vi "partsTracking.vi"(8 "error in (no error)":errorcluster, 11 "reference in":refnum<class "Project Panels.lvclass">=refnum) -> (0 "error out":errorcluster, 2 "saved?":bool, 3 "reference out":refnum<class "Project Panels.lvclass">)   [LabVIEW 2015, in "Project Panels.lvclass"]
uses:
  Project Panels.lvclass
  <vilib>/Utility/miscctls.llb/LVRowAndColumnTypeDef.ctl
  stateItem.ctl
  SYS/PartsTracking Controller_class/PartsTracking Controller.lvclass
  SYS/Notification Controller_class/Notification Controller.lvclass
panel:
  out "Cell Position":T1={"Row"=0, "Column"=4}
  out "title":string="Cosmed Asia Pacific - Parts Tracking"
  in  "partsTracking":string[][](table)
  out "statuBar":string="Stoped from User"
  in  "Save":bool
  in  "Stop Button":bool
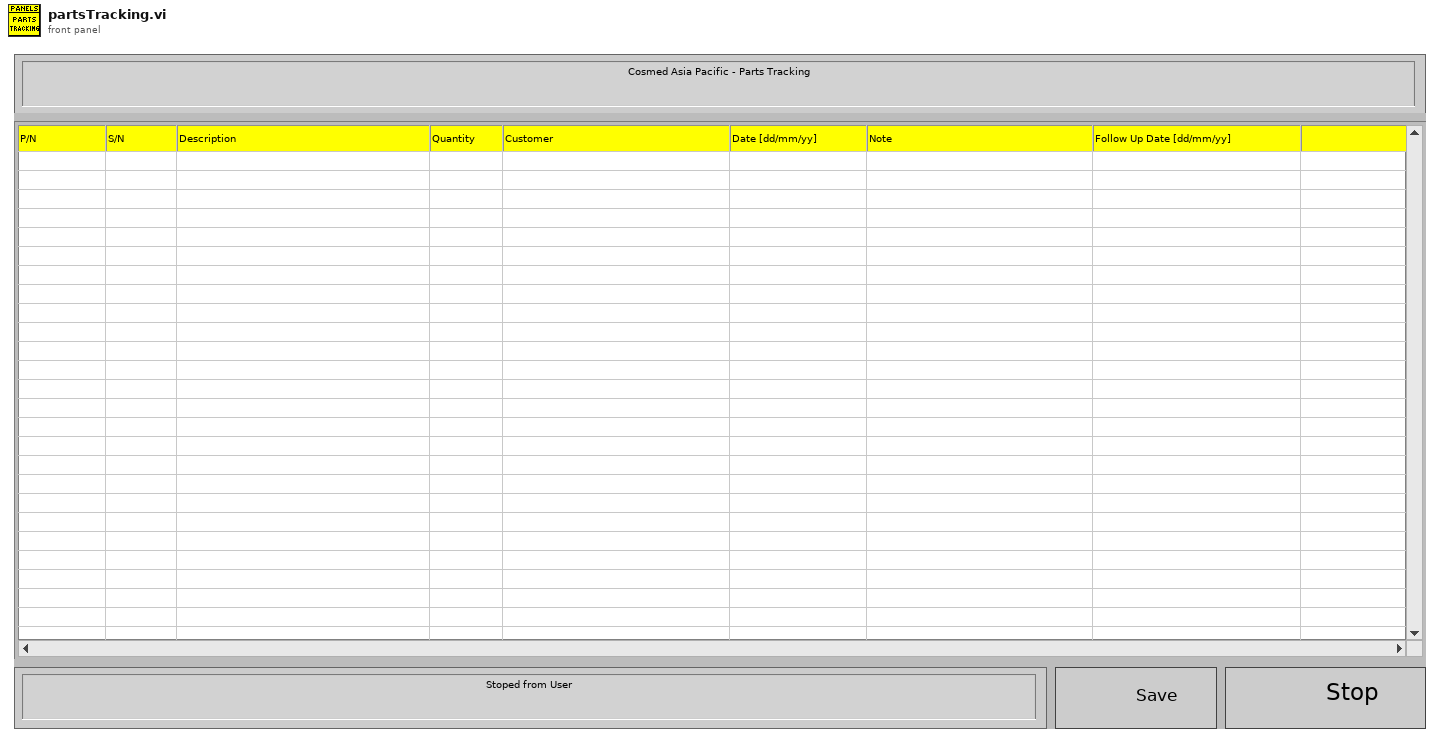
[diagram p1: front panel]
types:
  T1 = typedef "LVRowAndColumnTypeDef.ctl" = cluster{"Row":i32, "Column":i32}
  T2 = typedef "Project Panels.lvclass/stateItem.ctl" = enum16{"initiate", "waitEvent", "save", "search", "UploadFile", "nextItems", "stop"}
  T3 = typedef "Project Panels.lvclass/ObjectAttributesRef.ctl" = refnum<data-value>
  T4 = typedef "Project Panels.lvclass/ObjectAttributes.ctl" = cluster{"MyAttribute":dbl, "device_controller_ref":refnum<class "Devices Controller.lvclass">, "file_controller_ref":refnum<class "File Controller.lvclass">, "item_controller_ref":refnum<class "Items Controller.lvclass">, "item_tables":cluster{"checkIN":string[][], "checkOUT":string[][], "storage":string[][]}, "quickbook_table":cluster{"notes":string[][]}, "notification_controller_ref":refnum<class "Notification Controller.lvclass">, "partstracking_controller_ref":refnum<class "PartsTracking Controller.lvclass">, "product_tables":cluster{"k4b2":string[][], "fitmate":string[][], "RMR":string[][], "CPET":string[][], "BP":string[][], "PP":string[][], "k5":string[][], "bb-pft":string[][]}, "rowsColour":u32[]}
  T5 = typedef "LVPoint32TypeDef.ctl" = cluster{"Horizontal":i32, "Vertical":i32}
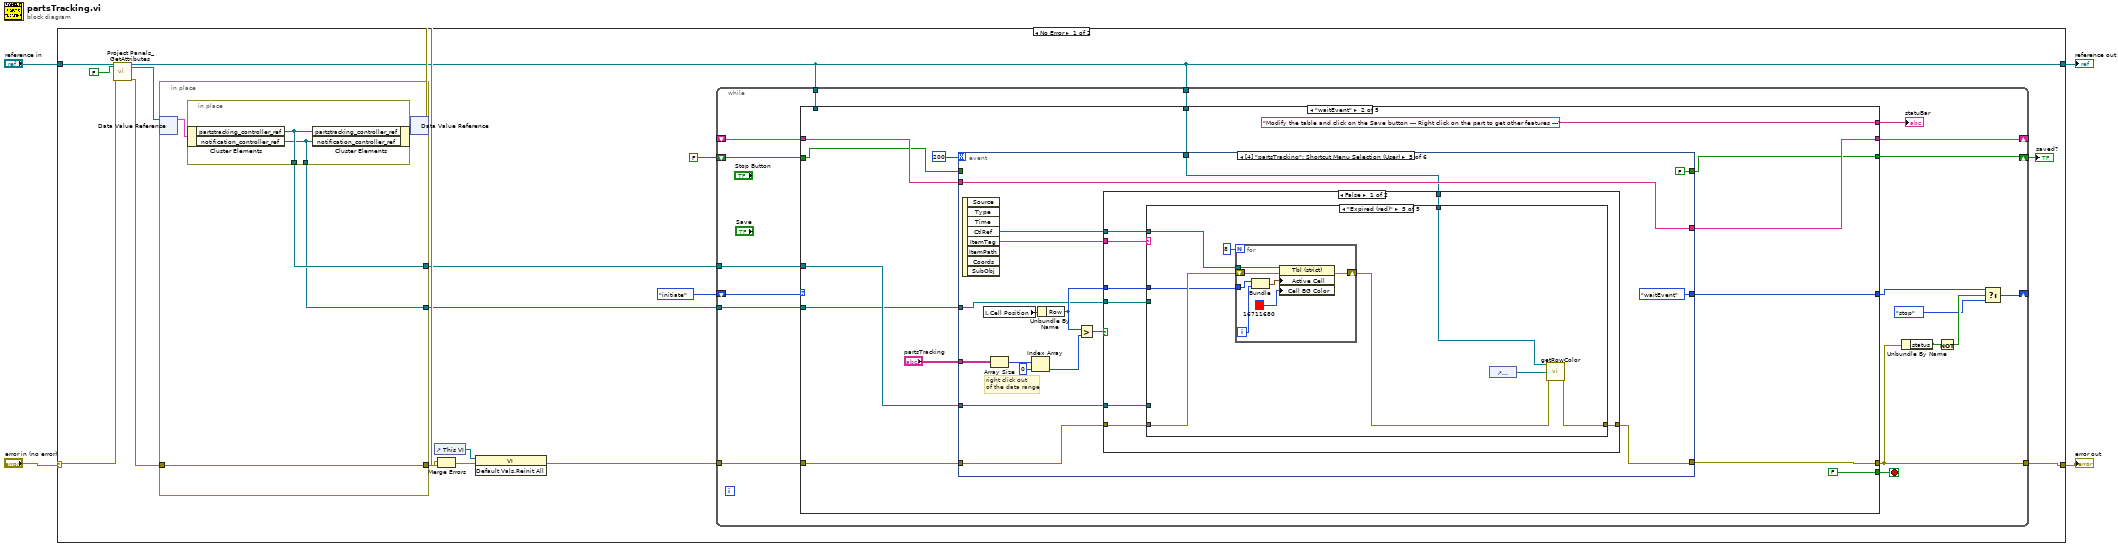
[diagram p0: block diagram]
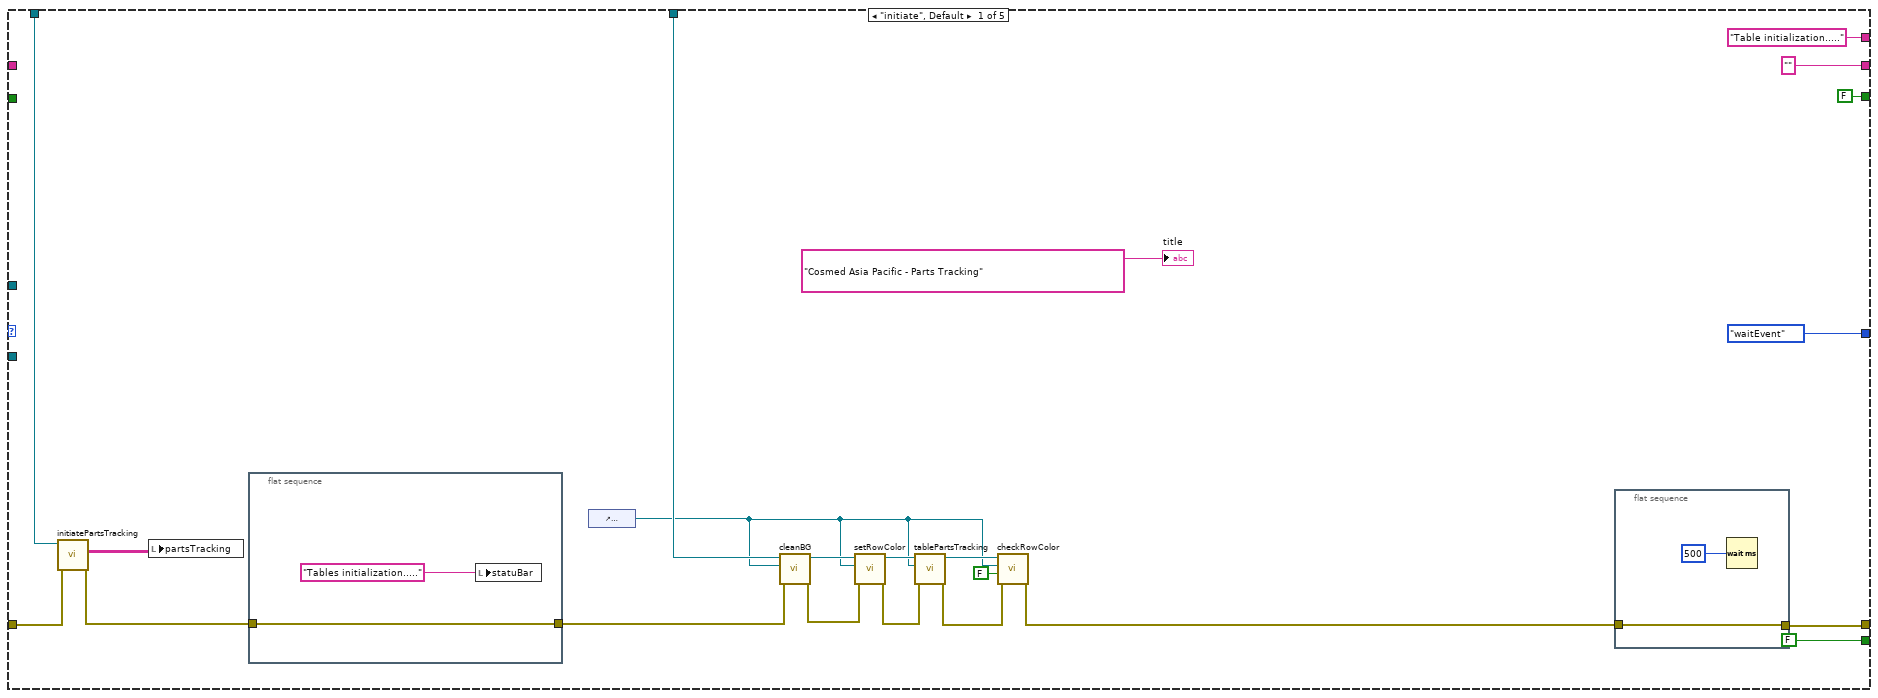
[diagram p2: hidden frame]
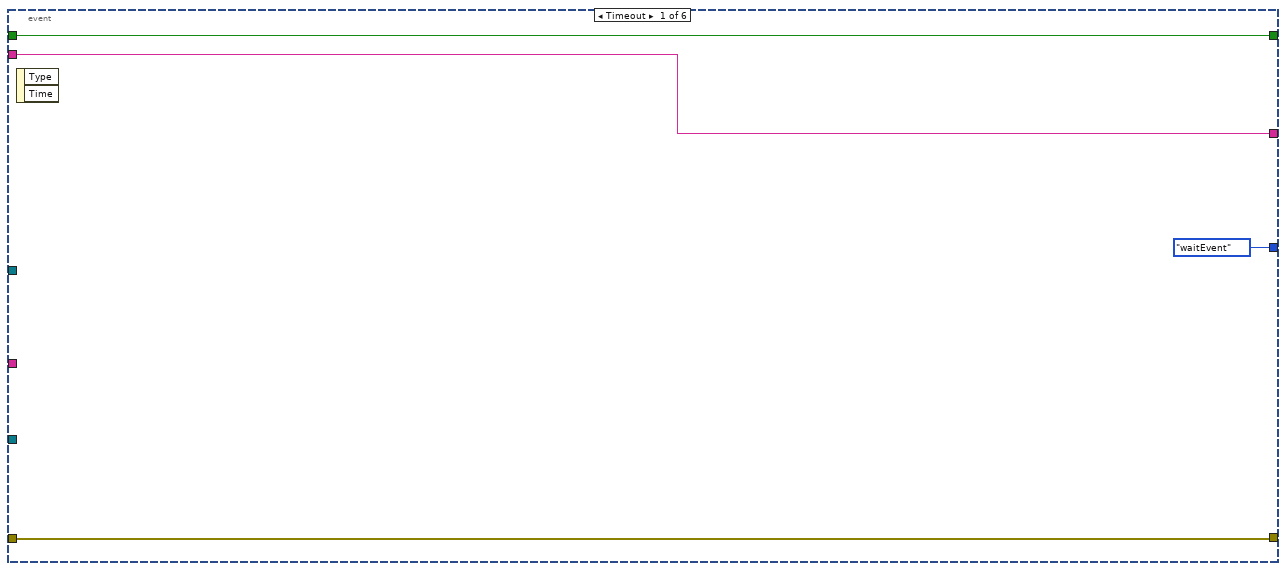
[diagram p3: hidden frame]
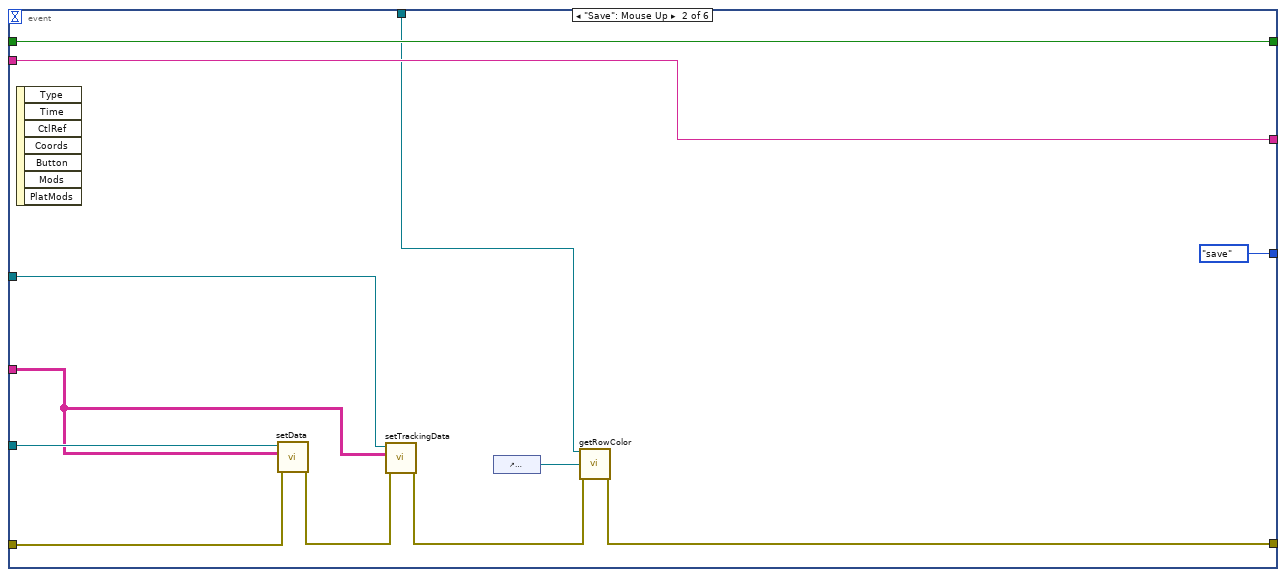
[diagram p4: hidden frame]
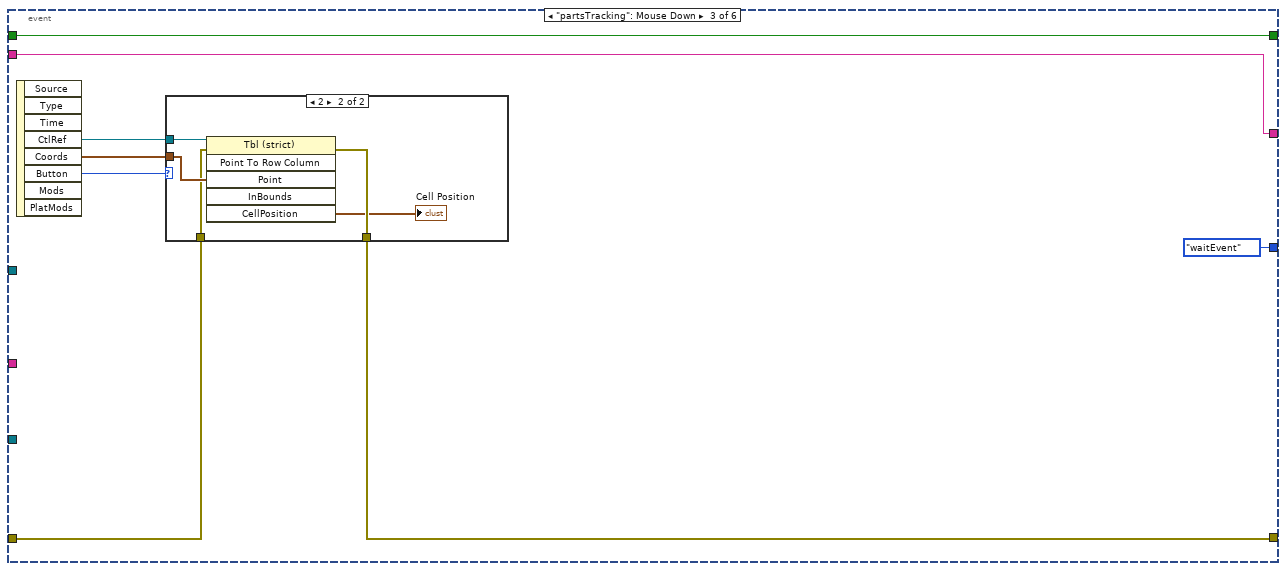
[diagram p5: hidden frame]
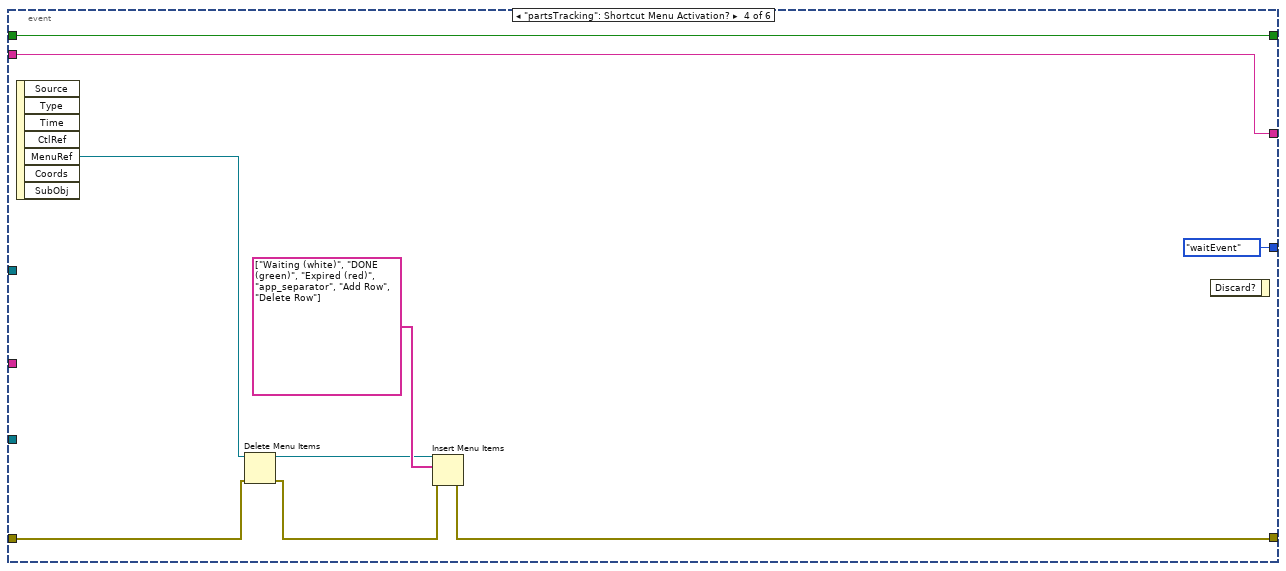
[diagram p7: hidden frame]
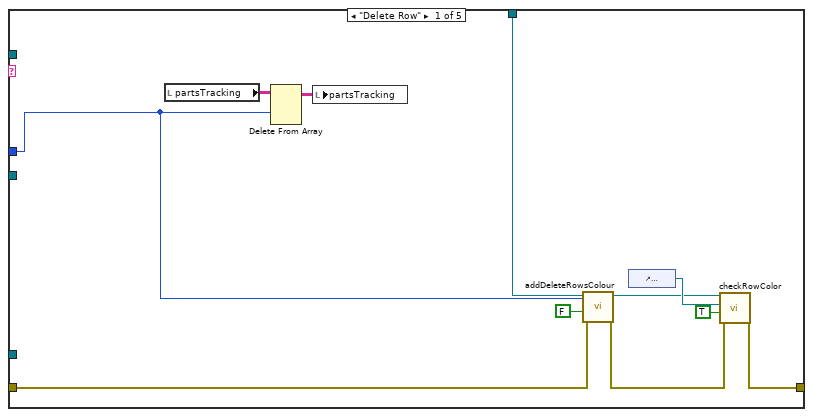
[diagram p8: hidden frame]
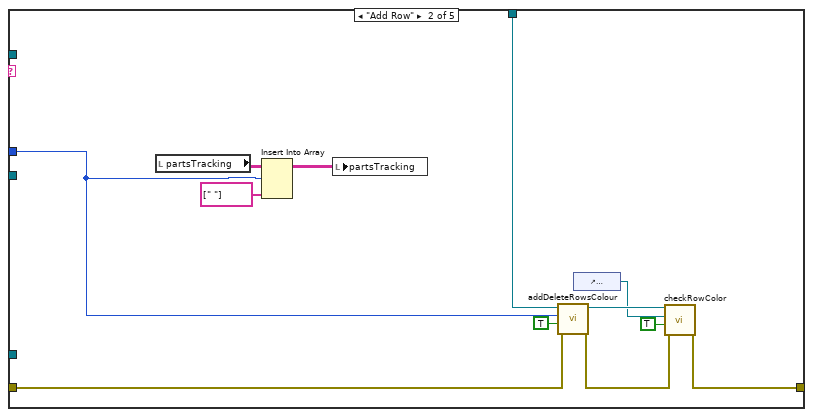
[diagram p9: hidden frame]
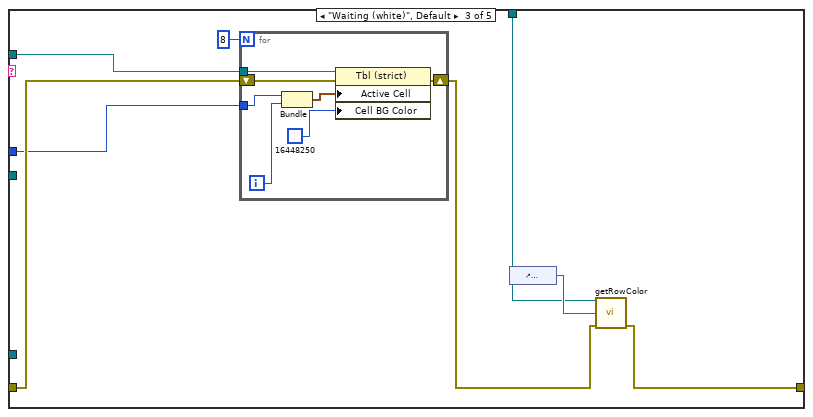
[diagram p10: hidden frame]
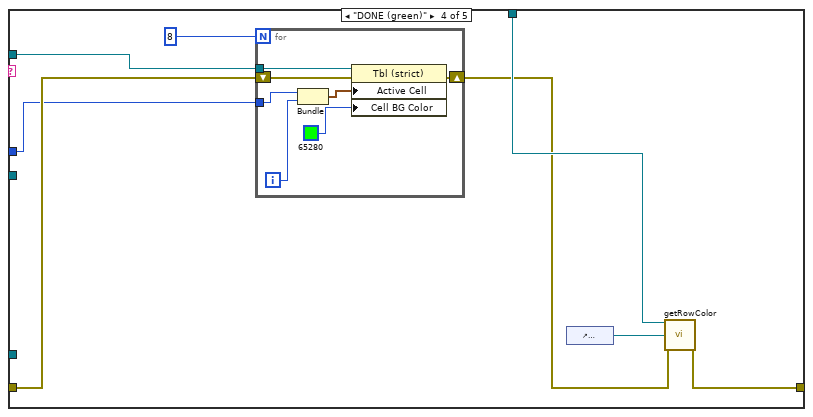
[diagram p11: hidden frame]
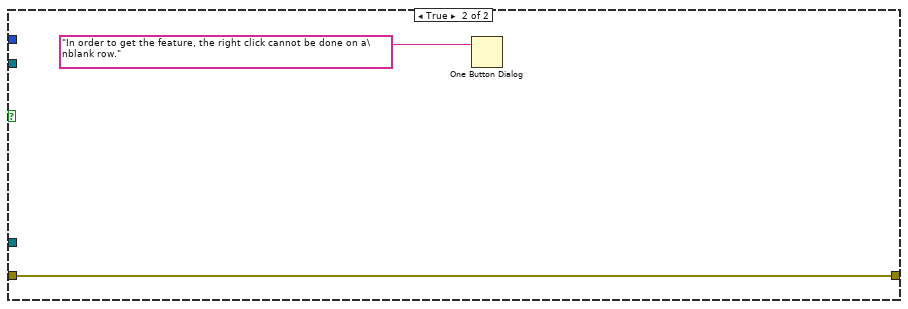
[diagram p12: hidden frame]
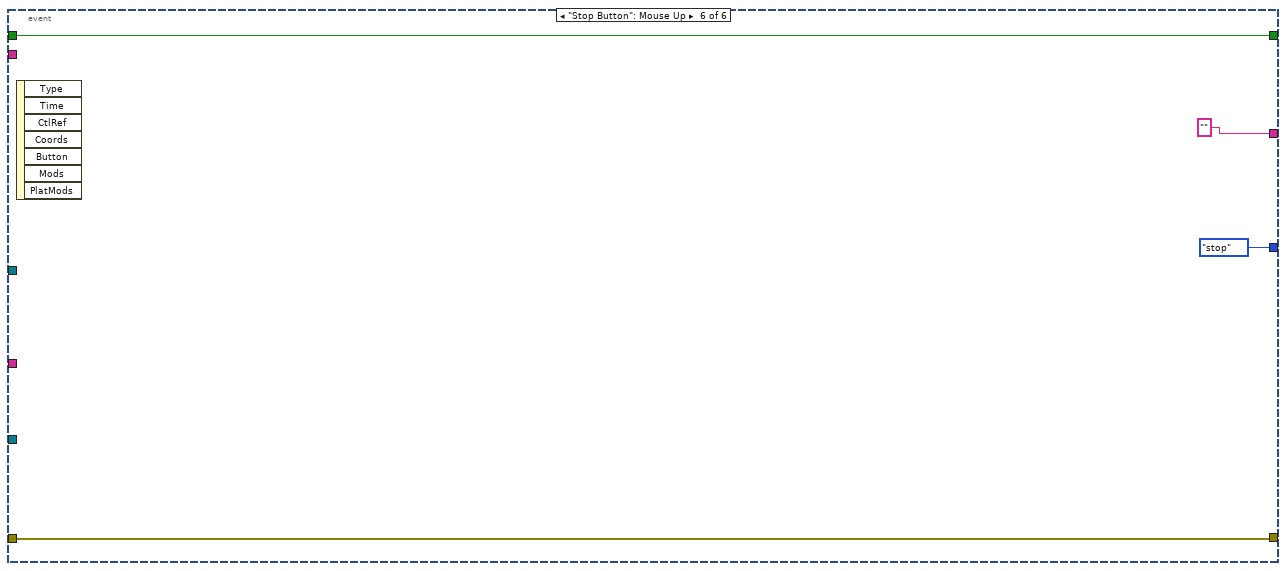
[diagram p13: hidden frame]
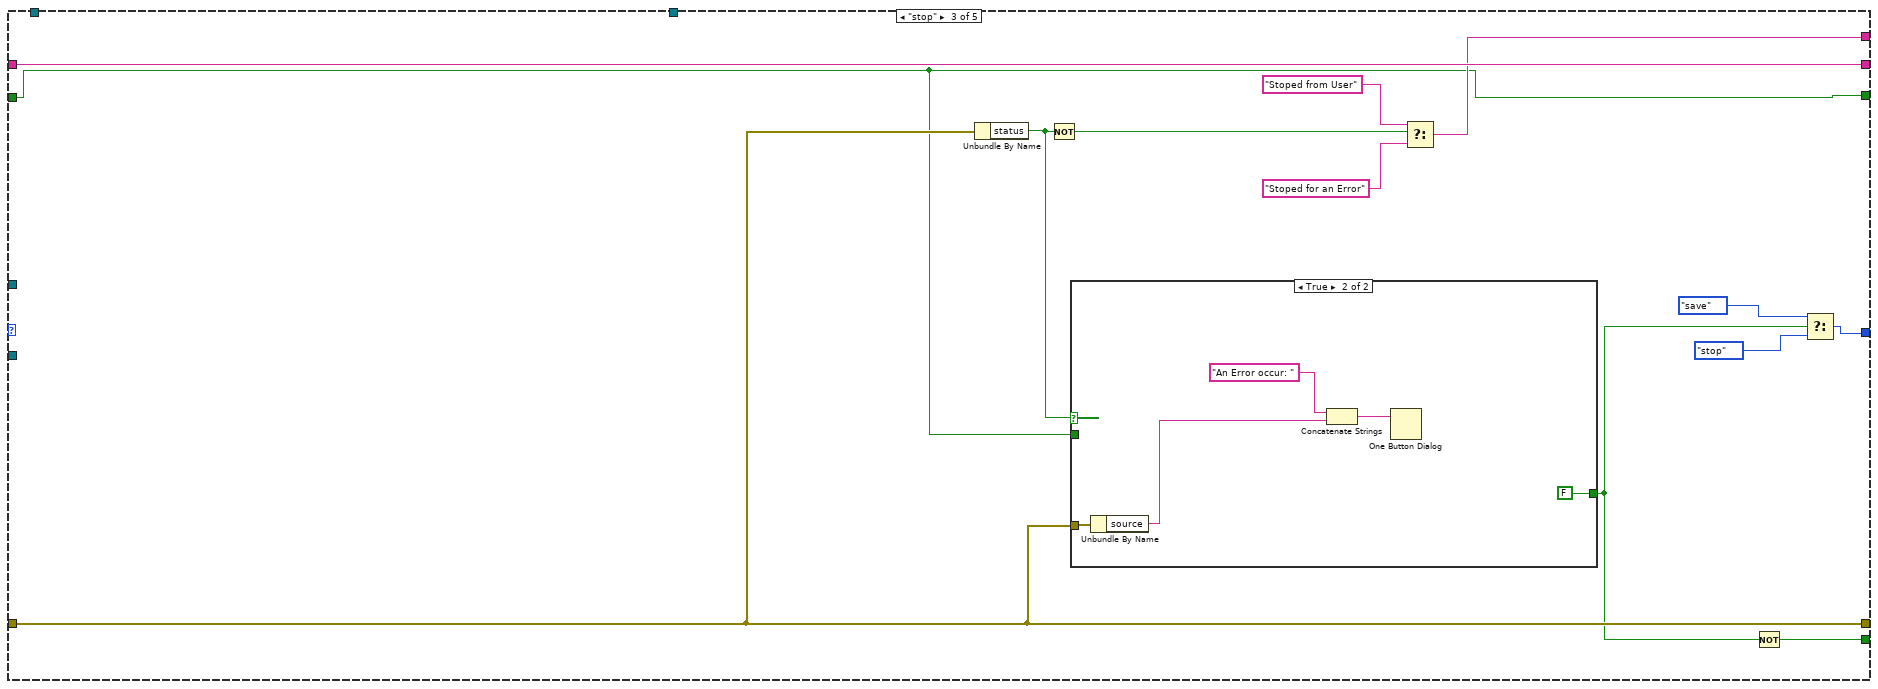
[diagram p14: hidden frame]
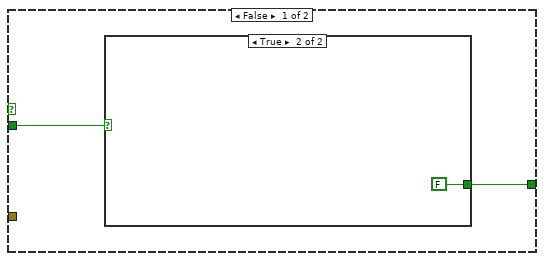
[diagram p15: hidden frame]
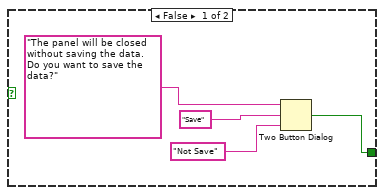
[diagram p16: hidden frame]
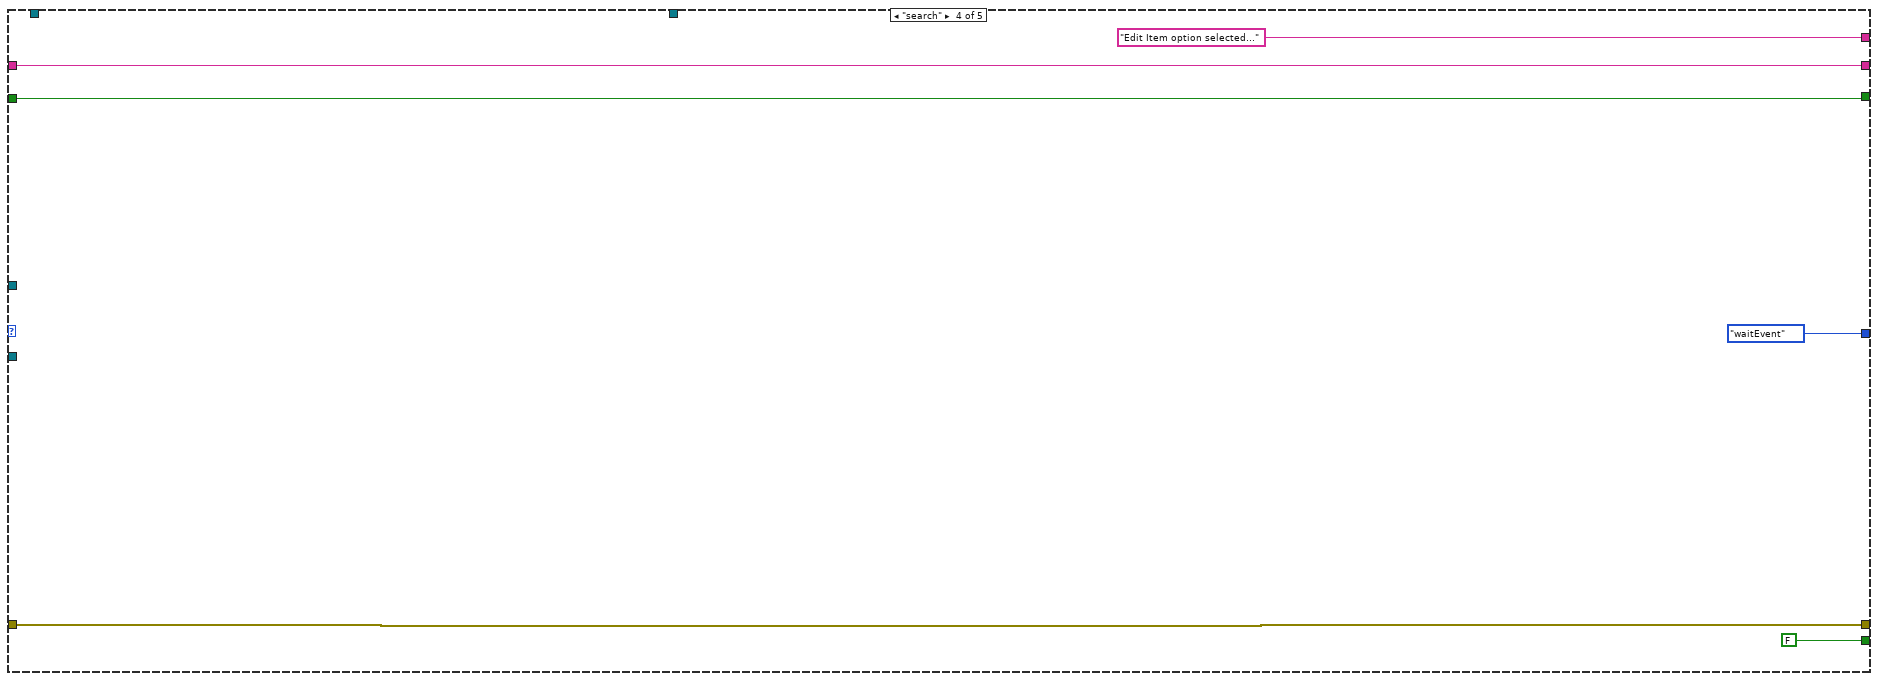
[diagram p17: hidden frame]
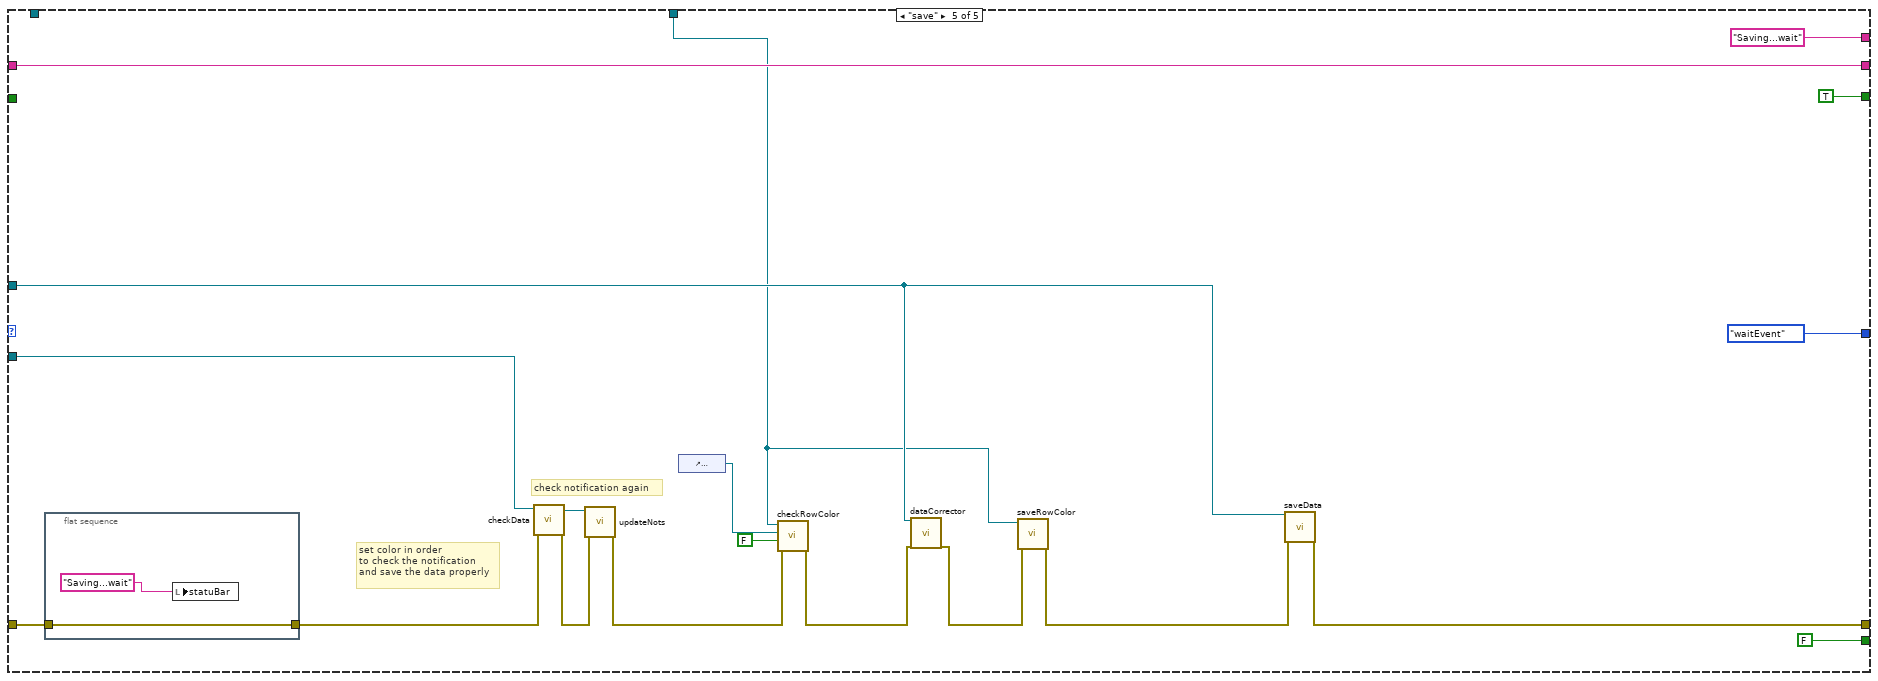
[diagram p18: hidden frame]
diagram:
  n1 = case shown="No Error" "error in (no error)" {
    selector: "error in (no error)" -> [w17 w278]
    tunnel: [w14 w278] -> w3
    tunnel: [w12 w277] -> w1
    tunnel: "reference in" -> [w19 w277]
    frame No Error {
      n2 = call "Project Panels_GetAttributes.vi"("reference in"=w19, "return data? (T)"=FALSE, "error in (no error)"=w17) -> ("reference out"=w12:refnum<class "Project Panels.lvclass">, "attributes ref"=w15:T3, "error out"=w16:errorcluster)  [unwired: 13 in, 1 out]
      n3 = in-place {
        in-place-border: w16 -> [w272]
        in-place-border: [w272] -> w20
        in-place-border: [w271] -> w10
        in-place-border: [w270] -> w6
        n4 = in-place-dvr #1(w15) -> (w273:T4)  [unwired: 1 out]
        n5 = in-place {
          in-place-border: [w276] -> w271
          in-place-border: [w275] -> w270
          n6 = in-place-cluster #2(w273) -> ("partstracking_controller_ref"=w276:refnum<class "PartsTracking Controller.lvclass">, "notification_controller_ref"=w275:refnum<class "Notification Controller.lvclass">)
          n7 = in-place-cluster #2("partstracking_controller_ref"=w276, "notification_controller_ref"=w275) -> (w274:T4)
        }
        n8 = in-place-dvr #1(w274) -> (w21:errorcluster)  [unwired: 1 out]
      }
      n9 = control-ref of="This VI"() -> (w11:refnum<vi>)
      n10 = Merge Errors(w20, w21) -> (w7:errorcluster)
      n11 = invoke class="VI" method="Default Vals.Reinit All"(reference=w11, error in=w7) -> (error out=w5:errorcluster)  [unwired: 1 in, 2 out]
      n12 = while {
        tunnel: w12 -> [w39]
        tunnel: w5 -> [w22]
        tunnel: [w37] -> w14
        shift-right: [w34] -> _
        shift-left: stateItem."initiate" ("state") -> [w38]
        shift-right: [w30] -> _
        shift-left: _ -> [w29]
        tunnel: w12 -> [w28]
        tunnel: w10 -> [w26]
        shift-right: [w24] -> w8
        shift-left: FALSE -> [w25]
        tunnel: w6 -> [w23]
        stop <- w32 stop-if-true
        n13 = case shown="\"waitEvent\"" w38 {
          tunnel: w39 -> [w45 w70 _ _ w251]
          tunnel: w22 -> [w54 w78 w221 w244 w263]
          tunnel: [w58 w73 w221 w244 w254] -> w37
          tunnel: [stateItem."waitEvent" ("state") w72 w223 stateItem."waitEvent" ("state") stateItem."waitEvent" ("state")] -> w35
          tunnel: [FALSE FALSE w218 FALSE FALSE] -> w32
          tunnel: ["Table initialization....." ("title") "Modify the table and click on the Save button --- Right click on the part to get other features ---" ("title") w227 "Edit Item option selected..." ("title") "Saving...wait" ("title")] -> w31
          tunnel: ["" w74 w230 w246 w265] -> w30
          tunnel: w29 -> [_ w75 w230 w246 w265]
          tunnel: w28 -> [w55 _ _ _ _]
          tunnel: w26 -> [_ w71 _ _ w257]
          tunnel: w25 -> [_ w68 w220 w243 _]
          tunnel: [FALSE w67 w220 w243 TRUE] -> w24
          tunnel: w23 -> [_ w69 _ _ w262]
          frame "initiate", Default {
            n14 = call "initiatePartsTracking.vi"("error in (no error)"=w54, "reference in"=w55) -> ("error out"=w53:errorcluster, "data"=w52:string[][])  [unwired: 7 in, 1 out]
            n15 = local write "partsTracking"(w52) -> ()
            n16 = flat-sequence {
              tunnel: w53 -> [w63]
              tunnel: [w63] -> w42
              frame #0 {
                n17 = local write "statuBar"("Tables initialization....." ("title")) -> ()
              }
            }
            n18 = control-ref of="partsTracking"() -> (w43:refnum<vi>)
            n19 = call "cleanBG.vi"("error in (no error)"=w42, "Table in"=w43, "reference in"=w45) -> ("error out"=w41:errorcluster, "reference out"=w44:refnum<class "Project Panels.lvclass">)  [unwired: 7 in]
            n20 = call "setRowColor.vi"("error in (no error)"=w41, "Table in"=w43, "reference in"=w44) -> ("error out"=w50:errorcluster, "reference out"=w51:refnum<class "Project Panels.lvclass">)  [unwired: 7 in]
            n21 = call "tablePartsTracking.vi"("error in (no error)"=w50, "Table in"=w43, "reference in"=w51) -> ("error out"=w48:errorcluster, "reference out"=w49:refnum<class "Project Panels.lvclass">)  [unwired: 7 in]
            n22 = call "checkRowColor.vi"("error in (no error)"=w48, "add/delete"=FALSE, "Table in"=w43, "reference in"=w49) -> ("error out"=w47:errorcluster)  [unwired: 6 in, 1 out]
            n23 = flat-sequence {
              tunnel: w47 -> [w65]
              tunnel: [w65] -> w58
              frame #0 {
                n24 = Wait (ms)(milliseconds to wait=u32 500) -> ()  [unwired: 1 out]
              }
            }
            "title" <- "Cosmed Asia Pacific - Parts Tracking" ("title")
          }
          frame "waitEvent" {
            n25 = event shown="[4] \"partsTracking\": Shortcut Menu Selection (User)" {
              selector: _ -> [_ _ _ _ _ _]
              dyn-events: _ -> [_ _ _ _ _ _]
              timeout: 200 -> [_ _ _ _ _ _]
              tunnel: w78 -> [w83 w93 w98 w116 w132 w217]
              tunnel: [w83 w85 w97 w113 w131 w217] -> w73
              tunnel: w75 -> [w82 w95 w101 w118 w135 _]
              tunnel: [w82 w95 w101 w118 w135 ""] -> w74
              tunnel: [stateItem."waitEvent" ("state") stateItem."save" ("state") stateItem."waitEvent" ("state") stateItem."waitEvent" ("state") stateItem."waitEvent" ("state") stateItem."stop" ("state")] -> w72
              tunnel: w71 -> [_ w92 _ _ w122 _]
              tunnel: w70 -> [_ w84 _ _ w119 _]
              tunnel: w69 -> [_ w90 _ _ w121 _]
              tunnel: w68 -> [w80 w89 w96 w110 _ w214]
              tunnel: [w80 w89 w96 w110 FALSE w214] -> w67
              tunnel: "partsTracking" -> [_ w88 _ _ w129 _]
              event Timeout {
                n26 = event-data() -> ()  [unwired: 1 in, 2 out]
              }
              event "Save": Mouse Up {
                n27 = event-data() -> ()  [unwired: 1 in, 7 out]
                n28 = call "setData.vi"("error in (no error)"=w93, "Data"=w88, "reference in"=w92) -> ("error out"=w91:errorcluster)  [unwired: 7 in, 1 out]
                n29 = call "setTrackingData.vi"("error in (no error)"=w91, "tracking_parts_data"=w88, "reference in"=w90) -> ("error out"=w86:errorcluster)  [unwired: 7 in, 1 out]
                n30 = control-ref of="partsTracking"() -> (w87:refnum<vi>)
                n31 = call "getRowColor.vi"("reference in"=w84, "Table in"=w87, "error in (no error)"=w86) -> ("error out"=w85:errorcluster)  [unwired: 11 in, 1 out]
              }
              event "partsTracking": Mouse Down {
                n32 = event-data() -> ("CtlRef"=w100:refnum<vi>, "Coords"=w99:T5, "Button"=w103:u16)  [unwired: 1 in, 5 out]
                n33 = case shown="2" w103 {
                  tunnel: w100 -> [_ w109]
                  tunnel: w99 -> [_ w108]
                  tunnel: w98 -> [w104 w107]
                  tunnel: [w104 w106] -> w97
                  frame 0, Default {
                  }
                  frame 2 {
                    n34 = invoke class="Tbl (strict)" method="Point To Row Column"(reference=w109, error in=w107, "Point"=w108) -> (error out=w106:errorcluster, "CellPosition"=→"Cell Position":T1)  [unwired: 3 in, 4 out]
                  }
                }
              }
              event "partsTracking": Shortcut Menu Activation? {
                n35 = event-data() -> ("MenuRef"=w115:refnum<k9>)  [unwired: 1 in, 6 out]
                n36 = Delete Menu Items(6:w116, 9:w115) -> (0:w114:errorcluster, 3:w111:refnum<k9>)  [unwired: 2 in]
                n37 = Insert Menu Items(6:w114, 8:string[] ["Waiting (white)", "DONE (green)", "Expired (red)", "app_separator", "Add Row", "Delete Row"] ("item names"), 9:w111) -> (0:w113:errorcluster)  [unwired: 3 in, 2 out]
                n38 = event-data() -> ()  [unwired: 2 in, 1 out]
              }
              event "partsTracking": Shortcut Menu Selection (User) {
                # "right click out\nof the data range"
                n39 = event-data() -> ("CtlRef"=w133:refnum<vi>, "ItemTag"=w134:string)  [unwired: 1 in, 6 out]
                n40 = local read "Cell Position"() -> (w126:T1)
                n41 = Array Size(array=w129) -> (size(s)=w128:i32[])
                n42 = Index Array(array=w128, index=0) -> (element=w125:i32)
                n43 = Unbundle By Name(w126) -> ("Row"=w123:i32)
                n44 = Greater?(x=w123, y=w125) -> (0:w124:bool)
                n45 = case shown="False" w124 {
                  tunnel: w134 -> [w143 _]
                  tunnel: w133 -> [w142 _]
                  tunnel: w132 -> [w141 w213]
                  tunnel: [w140 w213] -> w131
                  tunnel: w123 -> [w139 _]
                  tunnel: w122 -> [w138 _]
                  tunnel: w121 -> [w137 _]
                  tunnel: w119 -> [w136 _]
                  frame False {
                    n46 = case shown="\"Expired (red)\"" w143 {
                      tunnel: w142 -> [_ _ w174 w188 w203]
                      tunnel: w141 -> [w149 w161 w173 w187 w202]
                      tunnel: [w144 w157 w167 w182 w197] -> w140
                      tunnel: w139 -> [w150 w162 w171 w186 w201]
                      tunnel: w138 -> [_ _ _ _ _]
                      tunnel: w137 -> [_ _ _ _ _]
                      tunnel: w136 -> [w151 w163 w169 w184 w199]
                      frame "Delete Row" {
                        n47 = local read "partsTracking"() -> (w154:string[][])
                        n48 = Delete From Array(array=w154, index (row)=w150) -> (array with subset deleted=w153:string[][])  [unwired: 2 in, 1 out]
                        n49 = local write "partsTracking"(w153) -> ()
                        n50 = call "addDeleteRowsColour.vi"("error in (no error)"=w149, "Add?"=FALSE, "index"=w150, "reference in"=w151) -> ("error out"=w145:errorcluster, "reference out"=w146:refnum<class "Project Panels.lvclass">)  [unwired: 6 in]
                        n51 = control-ref of="partsTracking"() -> (w148:refnum<vi>)
                        n52 = call "checkRowColor.vi"("error in (no error)"=w145, "add/delete"=TRUE, "Table in"=w148, "reference in"=w146) -> ("error out"=w144:errorcluster)  [unwired: 6 in, 1 out]
                      }
                      frame "Add Row" {
                        n53 = local read "partsTracking"() -> (w166:string[][])
                        n54 = Insert Into Array(array=w166, index (row)=w162, new element=string[] [" "] ("new element/subarray")) -> (w164:string[][])  [unwired: 1 in]
                        n55 = local write "partsTracking"(w164) -> ()
                        n56 = call "addDeleteRowsColour.vi"("error in (no error)"=w161, "Add?"=TRUE, "index"=w162, "reference in"=w163) -> ("error out"=w158:errorcluster, "reference out"=w159:refnum<class "Project Panels.lvclass">)  [unwired: 6 in]
                        n57 = control-ref of="partsTracking"() -> (w156:refnum<vi>)
                        n58 = call "checkRowColor.vi"("error in (no error)"=w158, "add/delete"=TRUE, "Table in"=w156, "reference in"=w159) -> ("error out"=w157:errorcluster)  [unwired: 6 in, 1 out]
                      }
                      frame "Waiting (white)", Default {
                        n59 = for {
                          N: 8 -> [_]
                          tunnel: w174 -> [w181]
                          shift-right: [w179] -> w168
                          shift-left: w173 -> [w180]
                          tunnel: w171 -> [w177]
                          i -> [w176]
                          n60 = Bundle("Row"=w177, w176) -> (w175:cluster{"Row":i32, i32})  [unwired: 1 in]
                          n61 = property class="Tbl (strict)"(reference=w181, error in=w180, "Active Cell"=w175, "Cell BG Color"=u32 16448250) -> (error out=w179:errorcluster)  [unwired: 1 out]
                        }
                        n62 = control-ref of="partsTracking"() -> (w170:refnum<vi>)
                        n63 = call "getRowColor.vi"("reference in"=w169, "Table in"=w170, "error in (no error)"=w168) -> ("error out"=w167:errorcluster)  [unwired: 11 in, 1 out]
                      }
                      frame "DONE (green)" {
                        n64 = for {
                          N: 8 -> [_]
                          tunnel: w188 -> [w196]
                          shift-right: [w194] -> w183
                          shift-left: w187 -> [w195]
                          tunnel: w186 -> [w192]
                          i -> [w191]
                          n65 = Bundle("Row"=w192, w191) -> (w190:cluster{"Row":i32, i32})  [unwired: 1 in]
                          n66 = property class="Tbl (strict)"(reference=w196, error in=w195, "Active Cell"=w190, "Cell BG Color"=u32 65280) -> (error out=w194:errorcluster)  [unwired: 1 out]
                        }
                        n67 = control-ref of="partsTracking"() -> (w185:refnum<vi>)
                        n68 = call "getRowColor.vi"("reference in"=w184, "Table in"=w185, "error in (no error)"=w183) -> ("error out"=w182:errorcluster)  [unwired: 11 in, 1 out]
                      }
                      frame "Expired (red)" {
                        n69 = for {
                          N: 8 -> [_]
                          tunnel: w203 -> [w211]
                          shift-right: [w209] -> w198
                          shift-left: w202 -> [w210]
                          tunnel: w201 -> [w207]
                          i -> [w205]
                          n70 = Bundle("Row"=w207, w205) -> (w206:cluster{"Row":i32, i32})  [unwired: 1 in]
                          n71 = property class="Tbl (strict)"(reference=w211, error in=w210, "Active Cell"=w206, "Cell BG Color"=u32 16711680) -> (error out=w209:errorcluster)  [unwired: 1 out]
                        }
                        n72 = control-ref of="partsTracking"() -> (w200:refnum<vi>)
                        n73 = call "getRowColor.vi"("reference in"=w199, "Table in"=w200, "error in (no error)"=w198) -> ("error out"=w197:errorcluster)  [unwired: 11 in, 1 out]
                      }
                    }
                  }
                  frame True {
                    n74 = One Button Dialog(message="In order to get the feature, the right click cannot be done on a\nblank row.") -> ()  [unwired: 1 in, 1 out]
                  }
                }
              }
              event "Stop Button": Mouse Up {
                n75 = event-data() -> ()  [unwired: 1 in, 7 out]
              }
            }
          }
          frame "stop" {
            n76 = Unbundle By Name(w221) -> ("status"=w226:bool)
            n77 = Not(x=w226) -> (.not. x?=w225:bool)
            n78 = case shown="True" w226 {
              tunnel: w221 -> [_ w240]
              tunnel: [w232 FALSE ("Save")] -> w219
              tunnel: w220 -> [w231 _]
              frame False {
                n79 = case shown="True" w231 {
                  tunnel: [w235 FALSE ("Save")] -> w232
                  frame False {
                    n80 = Two Button Dialog(message="The panel will be closed without saving the data. Do you want to save the data?", 1:"Not Save" ("F button name (\"Cancel\")"), 2:"Save" ("T button name (\"OK\")")) -> (T button?=w235:bool)
                  }
                  frame True {
                  }
                }
              }
              frame True {
                n81 = Unbundle By Name(w240) -> ("source"=w239:string)
                n82 = Concatenate Strings("An Error occur: " ("message"), w239) -> (w242:string)
                n83 = One Button Dialog(message=w242) -> ()  [unwired: 1 in, 1 out]
              }
            }
            n84 = Select(t="Stoped from User" ("title"), s=w225, f="Stoped for an Error" ("title")) -> (s? t:f=w227:string)
            n85 = Not(x=w219) -> (.not. x?=w218:bool)
            n86 = Select(t=stateItem."save", s=w219, f=stateItem."stop" ("state")) -> (s? t:f=w223:T2)
          }
          frame "search" {
          }
          frame "save" {
            # "set color in order\nto check the notification\nand save the data properly"
            # "check notification again"
            n87 = flat-sequence {
              tunnel: w263 -> [w269]
              tunnel: [w269] -> w256
              frame #0 {
                n88 = local write "statuBar"("Saving...wait" ("title")) -> ()
              }
            }
            n89 = call "checkData.vi"("error in (no error)"=w256, "reference in"=w262) -> ("error out"=w260:errorcluster, "reference out"=w261:refnum<class "Notification Controller.lvclass">)  [unwired: 8 in]
            n90 = call "updateNots.vi"("error in (no error)"=w260, "reference in"=w261) -> ("error out"=w253:errorcluster)  [unwired: 8 in, 1 out]
            n91 = control-ref of="partsTracking"() -> (w258:refnum<vi>)
            n92 = call "checkRowColor.vi"("error in (no error)"=w253, "add/delete"=FALSE, "Table in"=w258, "reference in"=w251) -> ("error out"=w252:errorcluster)  [unwired: 6 in, 1 out]
            n93 = call "dataCorrector.vi"("reference in"=w257, "error in (no error)"=w252) -> ("error out"=w250:errorcluster)  [unwired: 16 in, 1 out]
            n94 = call "saveRowColor.vi"("error in (no error)"=w250, "reference in"=w251) -> ("error out"=w249:errorcluster)  [unwired: 8 in, 1 out]
            n95 = call "saveData.vi"("reference in"=w257, "error in (no error)"=w249) -> ("error out"=w254:errorcluster)  [unwired: 16 in, 1 out]
          }
        }
        "statuBar" <- w31
        n96 = Unbundle By Name(w37) -> ("status"=w36:bool)
        n97 = Not(x=w36) -> (.not. x?=w33:bool)
        n98 = Select(t=w35, s=w33, f=stateItem."stop" ("state")) -> (s? t:f=w34:T2)
      }
      "saved?" <- w8
    }
    frame Error {
    }
  }
  "error out" <- w3
  "reference out" <- w1
